vi "PH_Cont-601k_PSU.Set Readyness - Program.vi"(0 "VI in":refnum<vi>, 2 "Readyness - Program":T1, 5 "error in (no error)":errorcluster) -> (14 "VI out":refnum<vi>, 19 "error out":errorcluster)   [LabVIEW 2014, in "PH_Cont-601k_PSU.lvlib"]
uses:
  PH_Cont-601k_PSU.lvlib
  PH_Cont-601k_PSU.Readyness Program.ctl
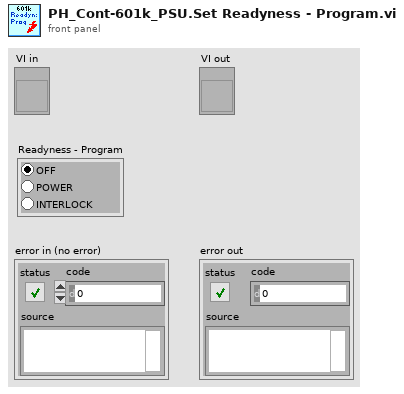
[diagram p1: front panel]
types:
  T1 = typedef "PH_Cont-601k_PSU.lvlib/PH_Cont-601k_PSU.Readyness Program.ctl" = enum32{"OFF", "POWER", "INTERLOCK"}
  T2 = typedef "PH_Cont-601k_PSU.lvlib/PH_Cont-601k_PSU.i attribute.ctl" = cluster{"GUI Refs":T3, "Interlock":bool, "Service ID applied Voltage":i32, "Device Settings":cluster{"Configuration":T4, "Flash Interval [s]":dbl, "Mode":T5, "Voltage [V]":u16, "Charge":bool, "VISA resource name":refnum<visa-resource-name>}, "Readyness":T6, "Information":cluster{"VISA resource name":refnum<visa-resource-name>, "Tagname Power On":string, "Interlock":cluster{"Instance":string, "Tagname":string}, "Limits [V]":cluster{"Lower":dbl, "Upper":dbl}, "Tagname PSU On":string}, "R2S":bool, "Charge is allowed":bool}
  T3 = typedef "PH_Cont-601k_PSU.lvlib/PH_Cont-601k_PSU.GUI Refs.ctl" = cluster{"Power On":refnum<vi>, "Hard- and Software":refnum<vi>, "Device Status":refnum<vi>, "Device Error":refnum<vi>, "Configuration":refnum<vi>, "Flash Interval [s]":refnum<vi>, "Interlock":refnum<vi>, "Interlock Indicator":refnum<vi>, "Voltage [V]":refnum<vi>, "Readyness":refnum<vi>, "Mode":refnum<vi>, "Reset Error":refnum<vi>, "Expert working":refnum<vi>, "Charge":refnum<vi>, "PSU On":refnum<vi>}
  T4 = typedef "PH_Cont-601k_PSU.lvlib/PH_Cont-601k_PSU.Configuration.ctl" = u16
  T5 = typedef "PH_Cont-601k_PSU.lvlib/PH_Cont-601k_PSU.Mode.ctl" = enum32{"STOP", "STANDBY", "READY", "EMISSION", "ERROR"}
  T6 = typedef "PH_Cont-601k_PSU.lvlib/PH_Cont-601k_PSU.Readyness.ctl" = cluster{"Program":T1, "Device":T7}
  T7 = typedef "PH_Cont-601k_PSU.lvlib/PH_Cont-601k_PSU.Readyness Device.ctl" = enum32{"OFF", "CONNECTING", "CONNECTED", "OPERATING", "EOC", "ERROR"}
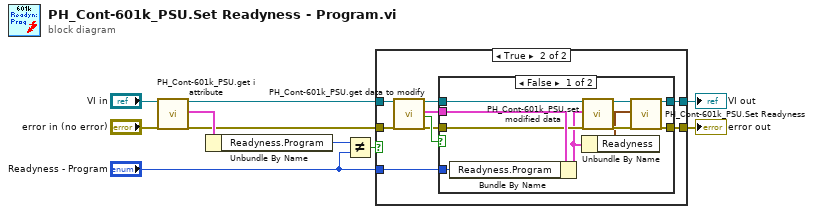
[diagram p0: block diagram]
diagram:
  n1 = call "PH_Cont-601k_PSU.get i attribute.vi"("i ref in"="VI in", "error in (no error)"="error in (no error)") -> ("i ref out"=w4:refnum<vi>, "i attribute"=w5:T2, "error out"=w3:errorcluster)  [unwired: 15 in]
  n2 = Unbundle By Name(w5) -> ("Readyness.Program"=w6:T1)
  n3 = Not Equal?(x=w6, y="Readyness - Program") -> (x != y?=w7:bool)
  n4 = case shown="True" w7 {
    tunnel: [w11 w21] -> w1
    tunnel: [w12 w13] -> w2
    tunnel: w3 -> [w11 w16]
    tunnel: w4 -> [w12 w15]
    tunnel: "Readyness - Program" -> [_ w14]
    frame False {
    }
    frame True {
      n5 = call "PH_Cont-601k_PSU.get data to modify.vi"("i ref in"=w15, "error in (no error)"=w16) -> ("i ref out"=w18:refnum<vi>, "i attribute"=w19:T2, "timed out"=w20:bool, "error out"=w17:errorcluster)  [unwired: 14 in]
      n6 = case shown="False" w20 {
        tunnel: [w25 w32] -> w21
        tunnel: w17 -> [w29 w32]
        tunnel: w18 -> [w31 w33]
        tunnel: [w27 w33] -> w13
        tunnel: w19 -> [w30 _]
        tunnel: w14 -> [w22 _]
        frame False {
          n7 = Bundle By Name(cluster=w30, "Readyness.Program"=w22) -> (w24:T2)
          n8 = Unbundle By Name(w24) -> ("Readyness"=w23:T6)
          n9 = call "PH_Cont-601k_PSU.set modified data.vi"("i ref in"=w31, "i attribute"=w24, "error in (no error)"=w29) -> ("i ref out"=w28:refnum<vi>, "error out"=w26:errorcluster)  [unwired: 15 in]
          n10 = call "PH_Cont-601k_PSU.Set Readyness.vi"("VI in"=w28, "Current Readyness"=w23, "error in (no error)"=w26) -> ("VI out"=w27:refnum<vi>, "error out"=w25:errorcluster)  [unwired: 15 in]
        }
        frame True {
        }
      }
    }
  }
  "error out" <- w1
  "VI out" <- w2
